vi "VerifyAcqStatus.vi"(8 "error in (no error)":errorcluster, 11 "S4GUI in":refnum<class "S4GUI.lvclass">) -> (0 "error out":errorcluster, 1 "all disabled":bool, 2 "idle":bool, 3 "S4GUI out":refnum<class "S4GUI.lvclass">)   [LabVIEW 2018, in "S4GUI.lvclass"]
uses:
  S4GUI.lvclass
  S4GUI.lvclass/S4GUI.ctl
  Acquisition/Acquisition.lvclass
  Channel/Channel.lvclass
panel:
  # "F : 1 ou mais canal habilitado\nT :  nenhum habilitado"
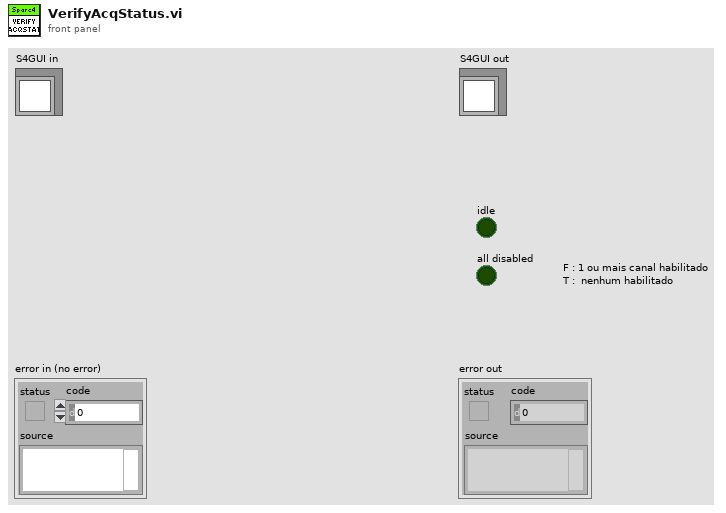
[diagram p1: front panel]
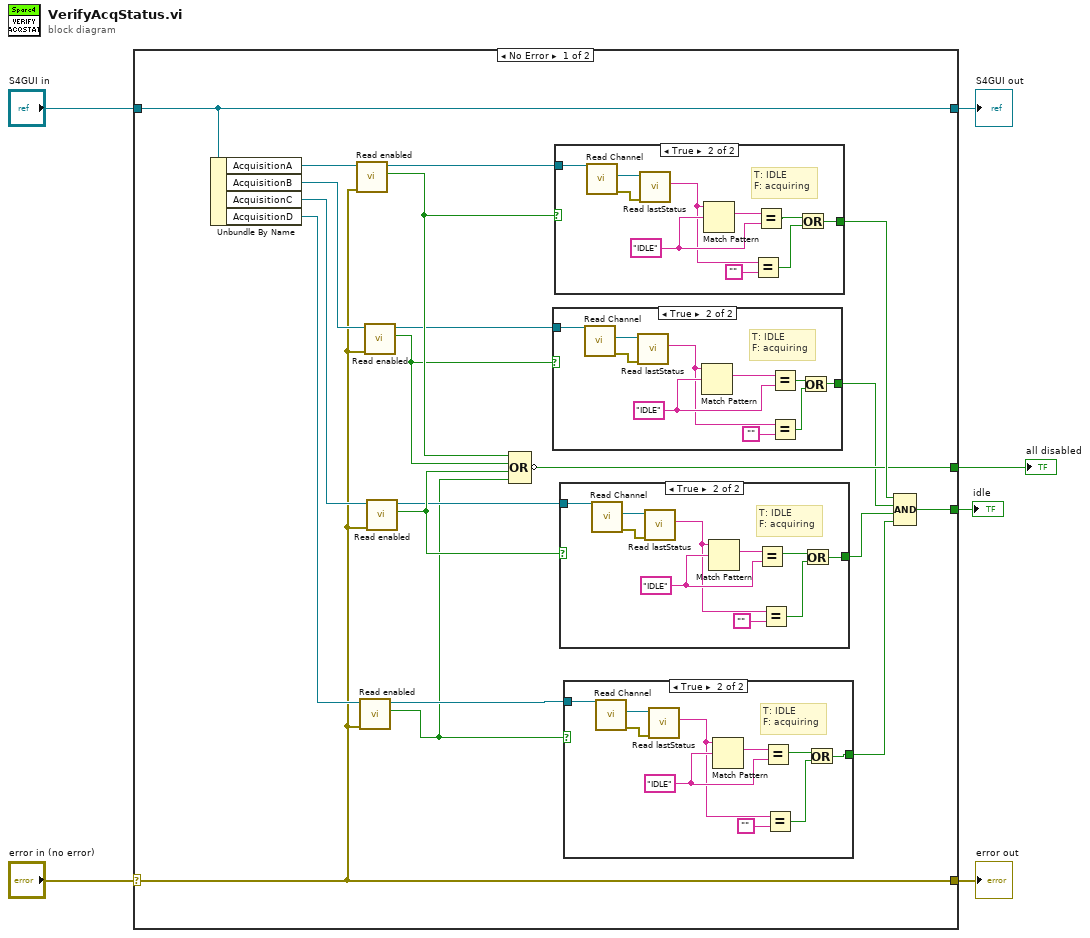
[diagram p0: block diagram]
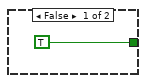
[diagram p2: hidden frame]
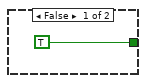
[diagram p3: hidden frame]
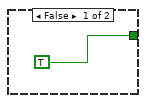
[diagram p4: hidden frame]
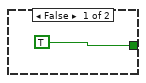
[diagram p5: hidden frame]
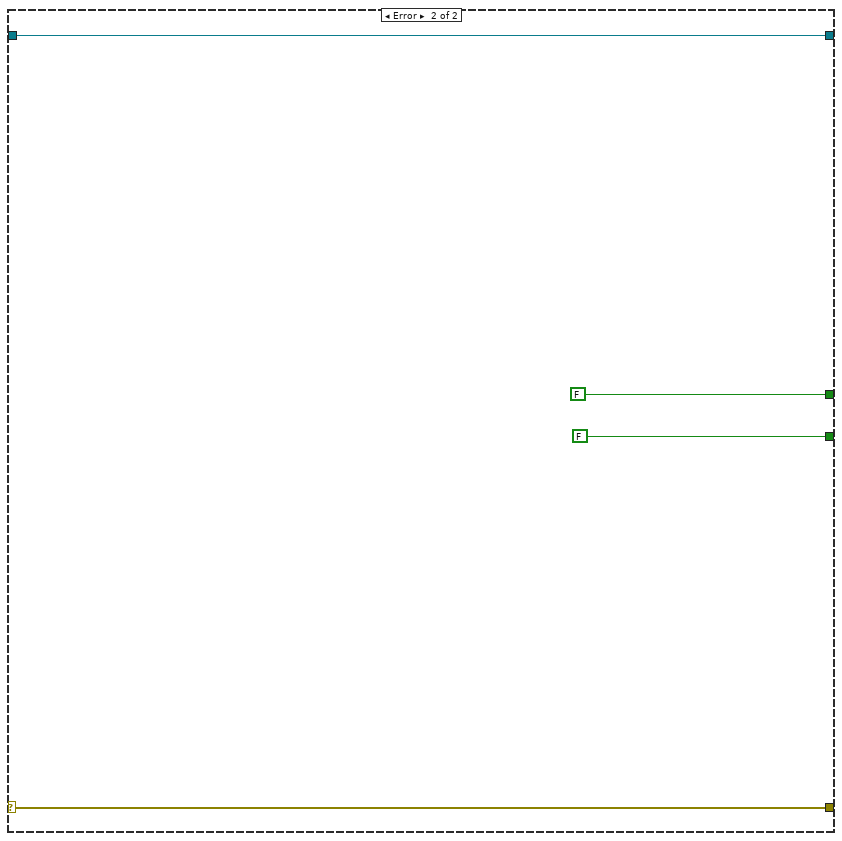
[diagram p6: hidden frame]
diagram:
  n1 = case shown="No Error" "error in (no error)" {
    selector: "error in (no error)" -> [w18 w74]
    tunnel: [w18 w74] -> w5
    tunnel: [w26 w73] -> w3
    tunnel: "S4GUI in" -> [w26 w73]
    tunnel: [w24 FALSE] -> w2
    tunnel: [w17 FALSE] -> w1
    frame No Error {
      n2 = Unbundle By Name(w26) -> ("AcquisitionA"=w23:refnum<class "Acquisition.lvclass">, "AcquisitionB"=w21:refnum<class "Acquisition.lvclass">, "AcquisitionC"=w20:refnum<class "Acquisition.lvclass">, "AcquisitionD"=w19:refnum<class "Acquisition.lvclass">)
      n3 = call-dynamic "Read enabled.vi"("error in (no error)"=w18, "Server in"=w23) -> ("enabled"=w16:bool, "Server out"=w22:refnum<class "Acquisition.lvclass">)  [unwired: 7 in, 1 out]
      n4 = call-dynamic "Read enabled.vi"("error in (no error)"=w18, "Server in"=w19) -> ("enabled"=w8:bool, "Server out"=w9:refnum<class "Acquisition.lvclass">)  [unwired: 7 in, 1 out]
      n5 = call-dynamic "Read enabled.vi"("error in (no error)"=w18, "Server in"=w21) -> ("enabled"=w14:bool, "Server out"=w15:refnum<class "Acquisition.lvclass">)  [unwired: 7 in, 1 out]
      n6 = call-dynamic "Read enabled.vi"("error in (no error)"=w18, "Server in"=w20) -> ("enabled"=w12:bool, "Server out"=w11:refnum<class "Acquisition.lvclass">)  [unwired: 7 in, 1 out]
      n7 = Compound Arithmetic op=OR(w16, w14, w12, w8) -> (invert w17:bool)
      n8 = case shown="True" w14 {
        tunnel: [TRUE w50] -> w13
        tunnel: w15 -> [_ w59]
        frame False {
        }
        frame True {
          w55 = "IDLE" ("regular expression")
          # "T: IDLE\nF: acquiring"
          n9 = call-dynamic "Read Channel.vi"("Acquisition in"=w59) -> ("error out"=w57:errorcluster, "Channel.lvclass"=w58:refnum<class "Channel.lvclass">)  [unwired: 8 in, 1 out]
          n10 = call-dynamic "Read lastStatus.vi"("error in (no error)"=w57, "Channel in"=w58) -> ("lastStatus"=w53:string)  [unwired: 7 in, 2 out]
          n11 = Match Pattern(string=w53, regular expression=w55) -> (match substring=w56:string)  [unwired: 1 in, 3 out]
          n12 = Equal?(x=w56, y=w55) -> (x = y?=w52:bool)
          n13 = Equal?(x=w53, y="") -> (x = y?=w51:bool)
          n14 = Or(x=w52, y=w51) -> (x .or. y?=w50:bool)
        }
      }
      n15 = case shown="True" w16 {
        tunnel: [TRUE w63] -> w25
        tunnel: w22 -> [_ w70]
        frame False {
        }
        frame True {
          w66 = "IDLE" ("regular expression")
          # "T: IDLE\nF: acquiring"
          n16 = call-dynamic "Read Channel.vi"("Acquisition in"=w70) -> ("error out"=w68:errorcluster, "Channel.lvclass"=w69:refnum<class "Channel.lvclass">)  [unwired: 8 in, 1 out]
          n17 = call-dynamic "Read lastStatus.vi"("error in (no error)"=w68, "Channel in"=w69) -> ("lastStatus"=w65:string)  [unwired: 7 in, 2 out]
          n18 = Match Pattern(string=w65, regular expression=w66) -> (match substring=w67:string)  [unwired: 1 in, 3 out]
          n19 = Equal?(x=w65, y="") -> (x = y?=w61:bool)
          n20 = Equal?(x=w67, y=w66) -> (x = y?=w62:bool)
          n21 = Or(x=w62, y=w61) -> (x .or. y?=w63:bool)
        }
      }
      n22 = case shown="True" w12 {
        tunnel: [TRUE w39] -> w10
        tunnel: w11 -> [_ w48]
        frame False {
        }
        frame True {
          w44 = "IDLE" ("regular expression")
          # "T: IDLE\nF: acquiring"
          n23 = call-dynamic "Read Channel.vi"("Acquisition in"=w48) -> ("error out"=w46:errorcluster, "Channel.lvclass"=w47:refnum<class "Channel.lvclass">)  [unwired: 8 in, 1 out]
          n24 = call-dynamic "Read lastStatus.vi"("error in (no error)"=w46, "Channel in"=w47) -> ("lastStatus"=w42:string)  [unwired: 7 in, 2 out]
          n25 = Match Pattern(string=w42, regular expression=w44) -> (match substring=w45:string)  [unwired: 1 in, 3 out]
          n26 = Equal?(x=w45, y=w44) -> (x = y?=w41:bool)
          n27 = Equal?(x=w42, y="") -> (x = y?=w40:bool)
          n28 = Or(x=w41, y=w40) -> (x .or. y?=w39:bool)
        }
      }
      n29 = case shown="True" w8 {
        tunnel: [TRUE w29] -> w7
        tunnel: w9 -> [_ w37]
        frame False {
        }
        frame True {
          w33 = "IDLE" ("regular expression")
          # "T: IDLE\nF: acquiring"
          n30 = call-dynamic "Read Channel.vi"("Acquisition in"=w37) -> ("error out"=w35:errorcluster, "Channel.lvclass"=w36:refnum<class "Channel.lvclass">)  [unwired: 8 in, 1 out]
          n31 = call-dynamic "Read lastStatus.vi"("error in (no error)"=w35, "Channel in"=w36) -> ("lastStatus"=w28:string)  [unwired: 7 in, 2 out]
          n32 = Match Pattern(string=w28, regular expression=w33) -> (match substring=w34:string)  [unwired: 1 in, 3 out]
          n33 = Equal?(x=w34, y=w33) -> (x = y?=w31:bool)
          n34 = Equal?(x=w28, y="") -> (x = y?=w30:bool)
          n35 = Or(x=w31, y=w30) -> (x .or. y?=w29:bool)
        }
      }
      n36 = Compound Arithmetic op=AND(w25, w13, w10, w7) -> (w24:bool)
    }
    frame Error {
    }
  }
  "error out" <- w5
  "S4GUI out" <- w3
  "idle" <- w2
  "all disabled" <- w1
